vi "from string.vi"(8 "error in":errorcluster, 9 "data":string, 10 "version":string, 11 "Digitizer Channel configuration":refnum<class "Digitizer Channel configuration.lvclass">) -> (0 "error out":errorcluster, 3 "Digitizer Channel configuration out":refnum<class "Digitizer Channel configuration.lvclass">)   [LabVIEW 2025, in "Digitizer.lvlib" / "Digitizer Channel configuration.lvclass"]
doc: "Provides an interface for loading a module configuration from a file or other serialized data source. It is recommended that all children of this class store data in two sets--data required for its own initialization, and any data required for parent initialization--and that each implementation uses the <b>Call Parent Method</b> primitive to de-serialize parent information.Copyright 2017 National Instruments Corporation\n\nLicensed under the Apache License, Version 2.0 (the \"License\"); you may not use this file except in compliance with the License. You may obtain a copy of the License at http://www.apache.org/licenses/LICENSE-2.0\nUnless required by applicable law or agreed to in writing, software distributed under the License is distributed on an \"AS IS\" BASIS, WITHOUT WARRANTIES OR CONDITIONS OF ANY KIND, either express or implied. See the License for the specific language governing permissions and limitations under the License."
uses:
  Digitizer Channel configuration.lvclass
  Digitizer Channel Setting.ctl
  Digitizer Channel configuration.lvclass/Digitizer Channel configuration.ctl
  Users/Public/Documents/Sandia National Labs/TSS Plugin/Abstract Engine.lvlibp/Channel configuration/Channel configuration.lvclass
  Users/Public/Documents/Sandia National Labs/TSS Plugin/CEF.lvlibp/serializable configuration/CEF_serializable configuration.lvclass
  Users/Public/Documents/Sandia National Labs/TSS Plugin/CEF.lvlibp
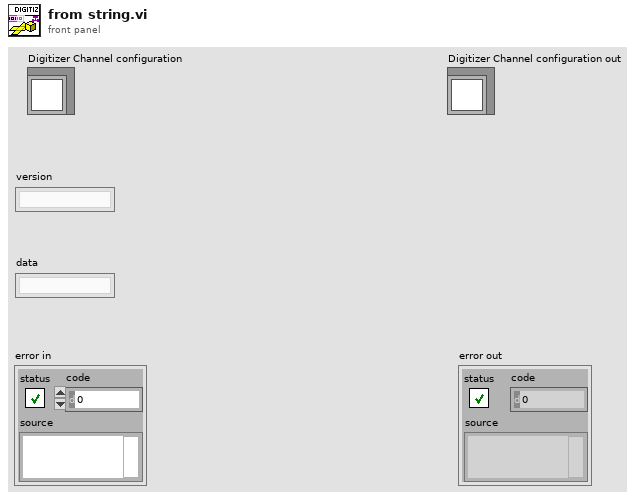
[diagram p1: front panel]
types:
  T1 = typedef "Digitizer.lvlib/Digitizer Channel configuration.lvclass/Digitizer Channel Setting.ctl" = cluster{"Max":dbl, "Min":dbl, "Data Reduction":string, "Averging Points":u32, "Decimate Interval":u32, "Aperture Options":cluster{"Tolerance":u32, "Burst":u32, "Min SampleRate":u32, "Min SampleIndex":u32}}
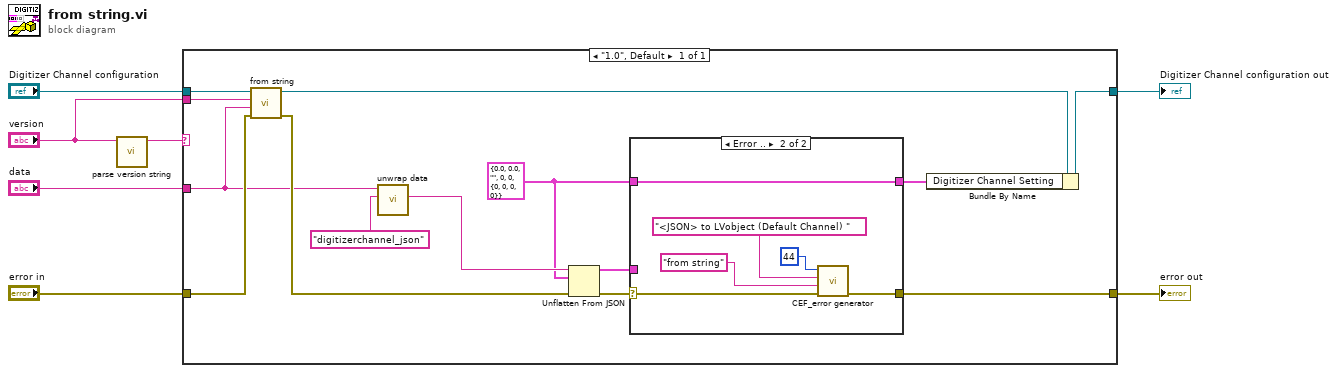
[diagram p0: block diagram]
diagram:
  n1 = call "parse version string.vi"("full version"="version") -> ("major.minor version"=w5:string)  [unwired: 7 in, 3 out]
  n2 = case shown="\"1.0\", Default" w5 {
    tunnel: "Digitizer Channel configuration" -> [w21]
    tunnel: [w16] -> w3
    tunnel: "data" -> [w13]
    tunnel: "error in" -> [w18]
    tunnel: "version" -> [w14]
    tunnel: [w8] -> w1
    frame "1.0", Default {
      w10 = T1 {"Max"=0.0, "Min"=0.0, "Data Reduction"="", "Averging Points"=0, "Decimate Interval"=0, "Aperture Options"={"Tolerance"=0, "Burst"=0, "Min SampleRate"=0, "Min SampleIndex"=0}} ("Setting")
      n3 = call-parent "from string.vi"("error in"=w18, "data"=w13, "version"=w14, "Channel configuration"=w21) -> ("error out"=w15:errorcluster, "Channel configuration out"=w20:refnum<class "Digitizer Channel configuration.lvclass">)  [unwired: 6 in]
      n4 = call "unwrap data.vi"("identifier"="digitizerchannel_json" ("additional identifier"), "data to unwrap"=w13) -> ("unwrapped data"=w17:string)  [unwired: 8 in, 1 out]
      n5 = Unflatten From JSON(JSON string=w17, type and defaults=w10, error in (no error)=w15) -> (value=w11:T1, error out=w12:errorcluster)  [unwired: 4 in]
      n6 = case shown="Error .." w12 {
        selector: w12 -> [w22 w26]
        tunnel: w11 -> [w23 _]
        tunnel: [w23 w25] -> w9
        tunnel: w10 -> [_ w25]
        tunnel: [w22 w24] -> w8
        frame No Error {
        }
        frame Error {
          n7 = call "CEF_error generator.vi"("error in"=w26, "source"="from string" ("message"), "append error message"="<JSON> to LVobject (Default Channel) " ("message"), "error code (0)"=44) -> ("error out"=w24:errorcluster)  [unwired: 5 in]
        }
      }
      n8 = Bundle By Name(cluster=w20, "Digitizer Channel Setting"=w9) -> (w16:refnum<class "Digitizer Channel configuration.lvclass">)
    }
  }
  "error out" <- w1
  "Digitizer Channel configuration out" <- w3
